vi "ConfigureGroups.vi"(8 "error in (no error)":errorcluster, 9 "AssetNodes":T1[](array[typedef]), 10 "single point channels":T12[](array[typedef]), 11 "device":T13) -> (0 "error out":errorcluster, 3 "config":T17)   [LabVIEW 2017, in "ScanEngine.lvlib"]
uses:
  <vilib>/addons/InsightCM/Devices/Shared/Common/ScanEngine/ScanEngine.lvlib
  <vilib>/addons/InsightCM/Devices/Shared/Common/ScanEngine/controls/Configuration.ctl
  <vilib>/addons/InsightCM/Devices/Shared/Common/ScanEngine/controls/Group.ctl
  <vilib>/addons/InsightCM/Devices/Shared/Common/ScanEngine/controls/Channel.ctl
  <vilib>/Utility/Data Type/Type Definitions/Data Type.ctl
  <vilib>/addons/InsightCM/MessageBus/Base/controls/KeyValuePair.ctl
  <vilib>/addons/InsightCM/MessageBus/Base/controls/R2_Device.ctl
  <vilib>/addons/InsightCM/MessageBus/Base/controls/DeviceState.ctl
  <vilib>/addons/InsightCM/MessageBus/Base/controls/R2_DataGroup.ctl
  <vilib>/addons/InsightCM/MessageBus/Base/controls/OperatingState.ctl
  <vilib>/addons/InsightCM/MessageBus/Base/controls/Trigger.ctl
  <vilib>/addons/InsightCM/MessageBus/Base/controls/Condition.ctl
  <vilib>/addons/InsightCM/MessageBus/Base/controls/BurstModeTrigger.ctl
  <vilib>/addons/InsightCM/MessageBus/Base/controls/R2_Channel.ctl
  <vilib>/addons/InsightCM/MessageBus/Base/controls/Metric.ctl
  <vilib>/addons/InsightCM/MessageBus/Base/controls/AssetNode.ctl
  <vilib>/addons/InsightCM/MessageBus/Base/controls/AssetState.ctl
  <vilib>/addons/InsightCM/MessageBus/Base/controls/TrendAlarmRule.ctl
  <vilib>/addons/InsightCM/MessageBus/Base/controls/TrendAlarmLevel.ctl
  <vilib>/addons/InsightCM/MessageBus/Base/controls/AlarmAction.ctl
  <vilib>/addons/InsightCM/MessageBus/Base/controls/AssetNodeReference.ctl
  <vilib>/addons/InsightCM/MessageBus/Base/controls/R2_DeviceModel.ctl
  <vilib>/addons/InsightCM/MessageBus/Base/controls/Tag.ctl
  <vilib>/addons/InsightCM/Utilities/DeviceModelHelpers/DeviceModelHelpers.lvlib
  <vilib>/Utility/Data Type/NI_Data Type.lvlib
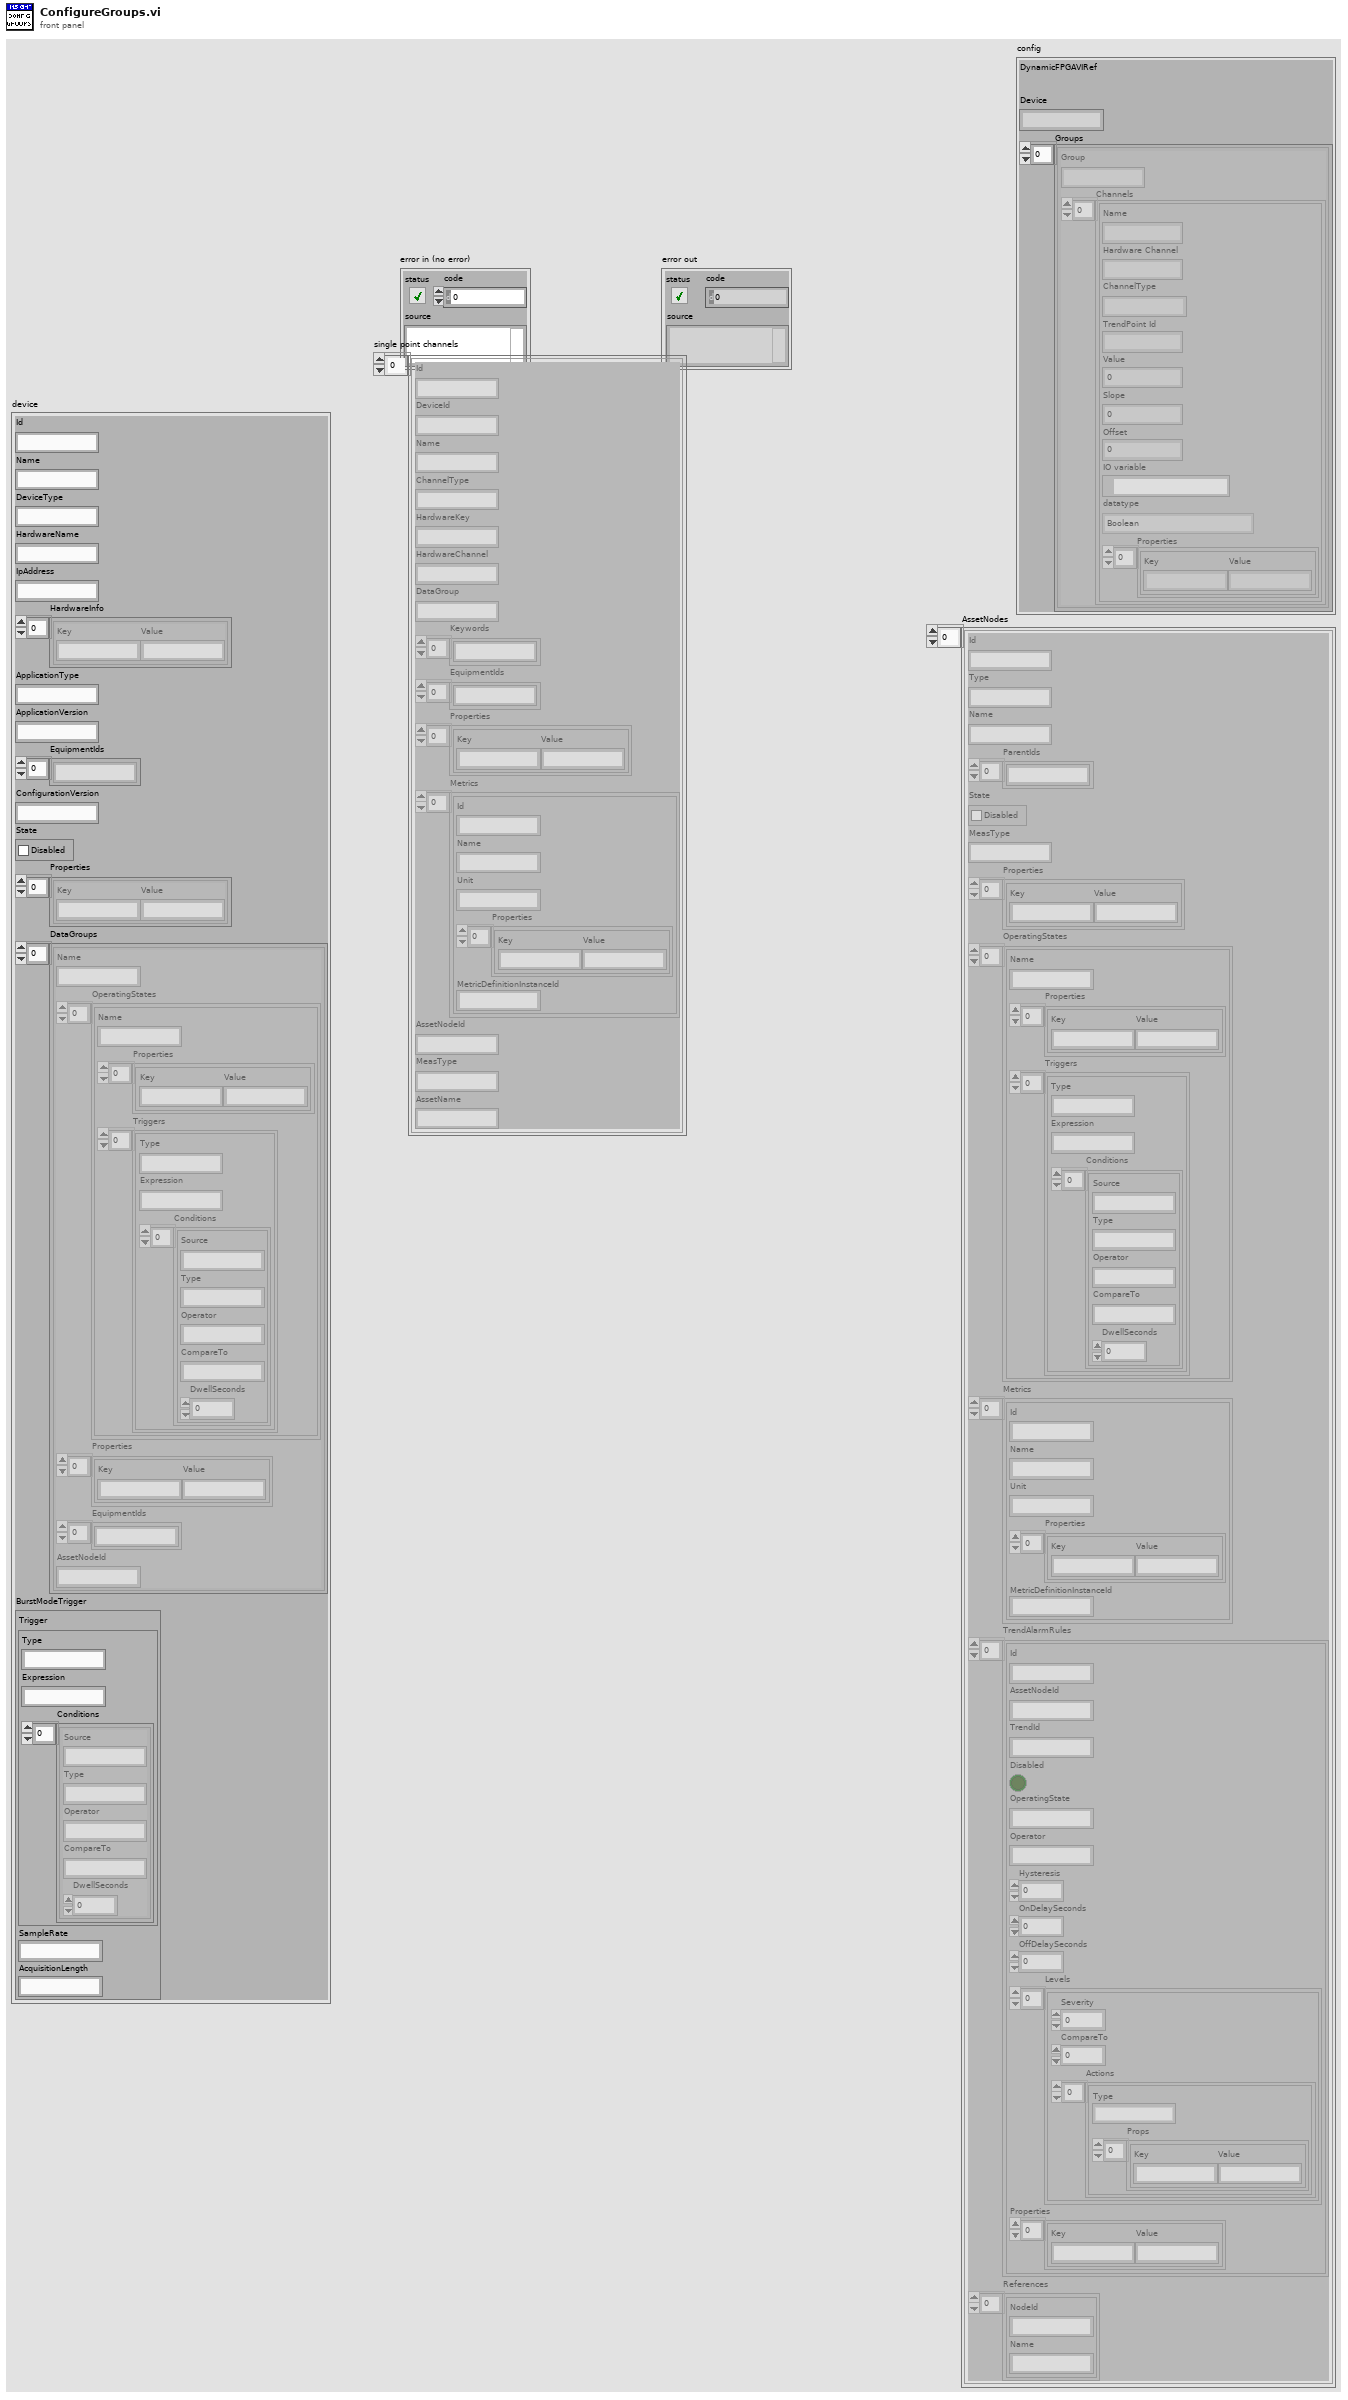
[diagram p1: front panel]
types:
  T1 = typedef "AssetNode.ctl" = cluster{"Id":string, "Type":string, "Name":string, "ParentIds":string[], "State":T2, "MeasType":string, "Properties":T3[], "OperatingStates":T4[], "Metrics":T7[], "TrendAlarmRules":T8[], "References":T11[]}
  T2 = typedef "AssetState.ctl" = cluster{"Disabled":bool}
  T3 = typedef "KeyValuePair.ctl" = cluster{"Key":string, "Value":string}
  T4 = typedef "OperatingState.ctl" = cluster{"Name":string, "Properties":T3[], "Triggers":T5[]}
  T5 = typedef "Trigger.ctl" = cluster{"Type":string, "Expression":string, "Conditions":T6[]}
  T6 = typedef "Condition.ctl" = cluster{"Source":string, "Type":string, "Operator":string, "CompareTo":string, "DwellSeconds":dbl}
  T7 = typedef "Metric.ctl" = cluster{"Id":string, "Name":string, "Unit":string, "Properties":T3[], "MetricDefinitionInstanceId":string}
  T8 = typedef "TrendAlarmRule.ctl" = cluster{"Id":string, "AssetNodeId":string, "TrendId":string, "Disabled":bool, "OperatingState":string, "Operator":string, "Hysteresis":dbl, "OnDelaySeconds":dbl, "OffDelaySeconds":dbl, "Levels":T9[], "Properties":T3[]}
  T9 = typedef "TrendAlarmLevel.ctl" = cluster{"Severity":i32, "CompareTo":dbl, "Actions":T10[]}
  T10 = typedef "AlarmAction.ctl" = cluster{"Type":string, "Props":T3[]}
  T11 = typedef "AssetNodeReference.ctl" = cluster{"NodeId":string, "Name":string}
  T12 = typedef "R2_Channel.ctl" = cluster{"Id":string, "DeviceId":string, "Name":string, "ChannelType":string, "HardwareKey":string, "HardwareChannel":string, "DataGroup":string, "Keywords":string[], "EquipmentIds":string[], "Properties":T3[], "Metrics":T7[], "AssetNodeId":string, "MeasType":string, "AssetName":string}
  T13 = typedef "R2_Device.ctl" = cluster{"Id":string, "Name":string, "DeviceType":string, "HardwareName":string, "IpAddress":string, "HardwareInfo":T3[], "ApplicationType":string, "ApplicationVersion":string, "EquipmentIds":string[], "ConfigurationVersion":string, "State":T14, "Properties":T3[], "DataGroups":T15[], "BurstModeTrigger":T16}
  T14 = typedef "DeviceState.ctl" = cluster{"Disabled":bool}
  T15 = typedef "R2_DataGroup.ctl" = cluster{"Name":string, "OperatingStates":T4[], "Properties":T3[], "EquipmentIds":string[], "AssetNodeId":string}
  T16 = typedef "BurstModeTrigger.ctl" = cluster{"Trigger":T5, "SampleRate":string, "AcquisitionLength":string}
  T17 = typedef "ScanEngine.lvlib/Configuration.ctl" = cluster{"DynamicFPGAVIRef":refnum<k20>, "Device":string, "Groups":T18[]}
  T18 = typedef "ScanEngine.lvlib/Group.ctl" = cluster{"Group":string, "Channels":T19[]}
  T19 = typedef "ScanEngine.lvlib/Channel.ctl" = cluster{"Name":string, "Hardware Channel":string, "ChannelType":string, "TrendPoint Id":string, "Value":sgl, "Slope":dbl, "Offset":dbl, "IO variable":refnum<k21>, "datatype":T20, "Properties":T3[]}
  T20 = typedef "NI_Data Type.lvlib/Data Type.ctl" = enum8{"Invalid Type", "Void", "I8", "I16", "I32", "I64", "U8", "U16", "U32", "U64", "Single Float", "Double Float", "Extended Float", "Single Complex", "Double Complex", "Extended Complex", "Enum U8", "Enum U16", "Enum U32", "Enum U64", "Single Float With Unit", "Double Float With Unit", "Extended Float With Unit", "Single Complex with Unit", "Double Complex with Unit", "Extended Complex with Unit", "Boolean", "String", "Path", "Picture", "Tag", "Array", "Cluster", "Variant", "LV Variant", "Waveform", "Timestamp", "Digital Waveform", "Digital Data", "ExpressData", "Refnum", "External Data", "VI", "Poly VI", "LabVIEW Class Instance", "Fixed Point"}
  T21 = typedef "R2_DeviceModel.ctl" = cluster{"Device":T13, "Channels":T12[], "Tags":T22[]}
  T22 = typedef "Tag.ctl" = cluster{"Id":string, "Path":string, "Name":string, "Datatype":string, "Props":T3[], "Keywords":string[]}
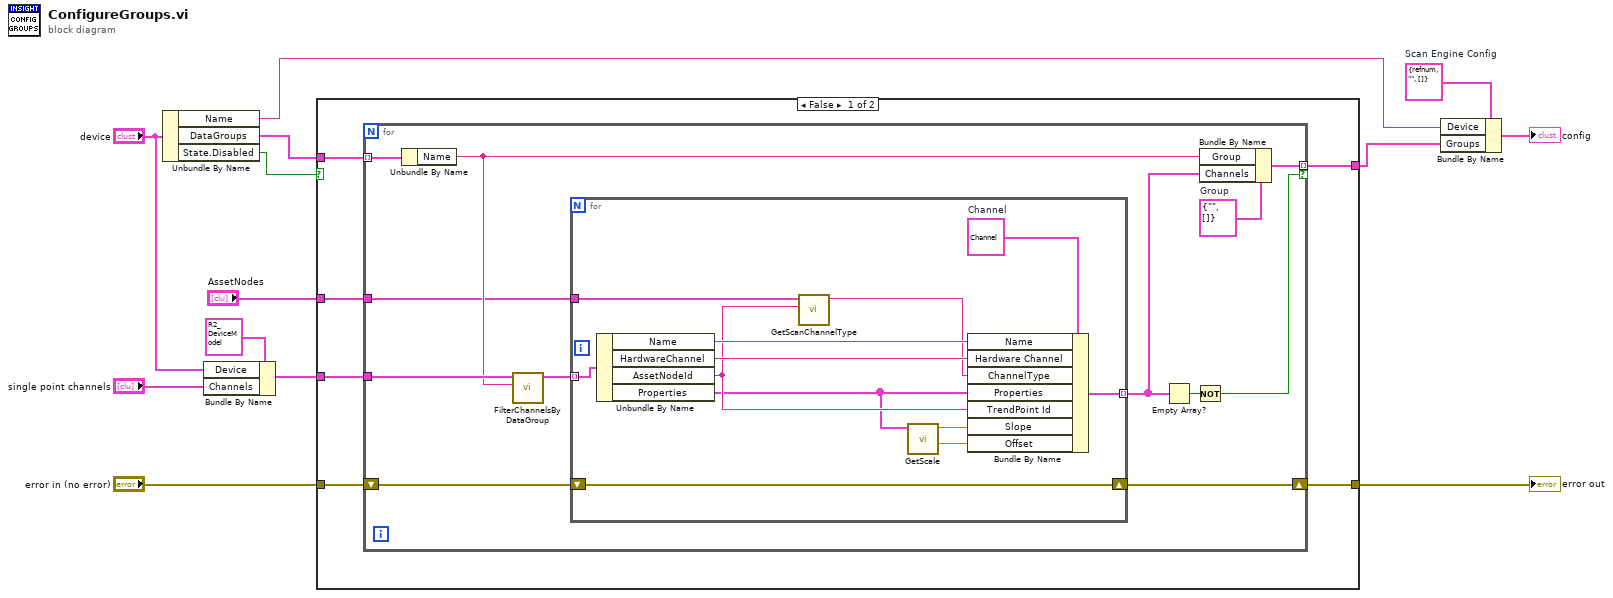
[diagram p0: block diagram]
diagram:
  w11 = T17 {"DynamicFPGAVIRef"=refnum, "Device"="", "Groups"=[]}  # Scan Engine Config
  n1 = Unbundle By Name("device") -> ("Name"=w7:string, "DataGroups"=w13:T15[], "State.Disabled"=w2:bool)
  n2 = Bundle By Name(cluster=T21 {"Device"={"Id"="", "Name"="", "DeviceType"="", "HardwareName"="", "IpAddress"="", "HardwareInfo"=[], "ApplicationType"="", "ApplicationVersion"="", "EquipmentIds"=[], "ConfigurationVersion"="", "State"={"Disabled"=FALSE}, "Properties"=[], "DataGroups"=[], "BurstModeTrigger"={"Trigger"={"Type"="", "Expression"="", "Conditions"=[]}, "SampleRate"="", "AcquisitionLength"=""}}, "Channels"=[], "Tags"=[]} ("device model"), "Device"="device", "Channels"="single point channels") -> (w4:T21)
  n3 = case shown="False" w2 {
    tunnel: w13 -> [w19 _]
    tunnel: [w18 w44] -> w12
    tunnel: [w17 _] -> w10
    tunnel: "error in (no error)" -> [w16 w44]
    tunnel: w4 -> [w15 _]
    tunnel: "AssetNodes" -> [w14 _]
    frame False {
      n4 = for {
        tunnel: w19 -> [w31] mode=indexing
        shift-right: [w30] -> w18
        shift-left: w16 -> [w27]
        tunnel: [w28] -> w17 mode=indexing if=w24
        tunnel: w15 -> [w23]
        tunnel: w14 -> [w20]
        w29 = T18 {"Group"="", "Channels"=[]}  # Group
        n5 = Unbundle By Name(w31) -> ("Name"=w21:string)
        n6 = call <vilib>:"FilterChannelsByDataGroup.vi"("group"=w21, "device model"=w23) -> ("channels in data group"=w22:T12[])  [unwired: 8 in, 1 out]
        n7 = for {
          shift-right: [w36] -> w30
          shift-left: w27 -> [w36]
          tunnel: [w43] -> w26 mode=indexing
          tunnel: w22 -> [w42] mode=indexing
          tunnel: w20 -> [w35]
          w41 = T19 {"Name"="", "Hardware Channel"="", "ChannelType"="", "TrendPoint Id"="", "Value"=0.0, "Slope"=0.0, "Offset"=0.0, "IO variable"="", "datatype"=enum."Invalid Type", "Properties"=[]}  # Channel
          n8 = Unbundle By Name(w42) -> ("Name"=w37:string, "HardwareChannel"=w40:string, "AssetNodeId"=w33:string, "Properties"=w32:T3[])
          n9 = call <vilib>:"GetScanChannelType.vi"("AssetNodeId"=w33, "AssetNodes"=w35) -> ("Type"=w34:string)  [unwired: 9 in]
          n10 = call <vilib>:"GetScale.vi"("Properties"=w32) -> ("offset"=w38:dbl, "slope"=w39:dbl)  [unwired: 9 in]
          n11 = Bundle By Name(cluster=w41, "Name"=w37, "Hardware Channel"=w40, "ChannelType"=w34, "Properties"=w32, "TrendPoint Id"=w33, "Slope"=w39, "Offset"=w38) -> (w43:T19)
        }
        n12 = Empty Array?(array=w26) -> (empty?=w25:bool)
        n13 = Not(x=w25) -> (.not. x?=w24:bool)
        n14 = Bundle By Name(cluster=w29, "Group"=w21, "Channels"=w26) -> (w28:T18)
      }
    }
    frame True {
    }
  }
  "error out" <- w12
  n15 = Bundle By Name(cluster=w11, "Device"=w7, "Groups"=w10) -> (→"config":T17)
